vi "AssertTimer.vi"() -> ()   [LabVIEW 2016, in "test_AssertTimer.lvlib"]
uses:
  test_AssertTimer.lvlib
  <vilib>/addons/_JKI Toolkits/Caraya/classes/Test/Test.lvclass
  main/apis/Assert/AssertTime/AssertTimer.lvlib
panel:
  out "error out":errorcluster
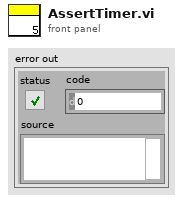
[diagram p1: front panel]
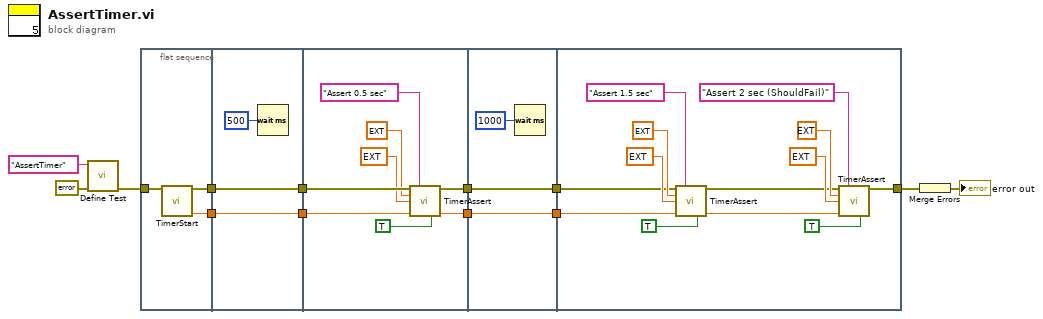
[diagram p0: block diagram]
diagram:
  n1 = call <vilib>:"Define Test.vi"("error in (no error)"=errorcluster {"status"=FALSE, "code"=0, "source"=""}, "Label (VI Title)"="AssertTimer") -> ("error out"=w11:errorcluster)  [unwired: 9 in]
  n2 = flat-sequence {
    tunnel: w11 -> [w16]
    tunnel: [w15] -> w10
    tunnel: [w14] -> w8
    tunnel: w10 -> [w19]
    tunnel: [w19] -> w9
    tunnel: w8 -> [w18]
    tunnel: [w18] -> w6
    tunnel: w9 -> [w27]
    tunnel: w6 -> [w25]
    tunnel: [w26] -> w5
    tunnel: [w20] -> w2
    tunnel: w5 -> [w30]
    tunnel: [w30] -> w4
    tunnel: [w28] -> w3
    tunnel: w2 -> [w28]
    tunnel: [w32] -> w7
    tunnel: w4 -> [w39]
    tunnel: w3 -> [w38]
    frame #0 {
      n3 = call "TimerStart.vi"("error in (no error)"=w16) -> ("error out"=w15:errorcluster, "StartTime"=w14:dbl)  [unwired: 13 in]
    }
    frame #1 {
      n4 = Wait (ms)(milliseconds to wait=u32 500) -> ()  [unwired: 1 out]
    }
    frame #2 {
      n5 = call "TimerAssert.vi"("error in (no error)"=w27, "Label"="Assert 0.5 sec", "Expected Time"=ext 0.5, "Tolerance"=ext 0.99, "Start Time in"=w25, "Use Percentage of X (F)"=TRUE) -> ("error out"=w26:errorcluster, "Start Time out"=w20:dbl)  [unwired: 8 in]
    }
    frame #3 {
      n6 = Wait (ms)(milliseconds to wait=u32 1000) -> ()  [unwired: 1 out]
    }
    frame #4 {
      n7 = call "TimerAssert.vi"("error in (no error)"=w39, "Label"="Assert 1.5 sec", "Expected Time"=ext 1.5, "Tolerance"=ext 0.99, "Start Time in"=w38, "Use Percentage of X (F)"=TRUE) -> ("error out"=w33:errorcluster, "Start Time out"=w31:dbl)  [unwired: 8 in]
      n8 = call "TimerAssert.vi"("error in (no error)"=w33, "Label"="Assert 2 sec (ShouldFail)", "Expected Time"=ext 2.0, "Tolerance"=ext 0.99, "Start Time in"=w31, "Use Percentage of X (F)"=TRUE) -> ("error out"=w32:errorcluster)  [unwired: 8 in, 1 out]
    }
  }
  n9 = Merge Errors(w7) -> (→"error out":errorcluster)
